vi "Untitled 7.vi"(0 "Tree":string(tree), 2 "Folder_Path":path=path "D:/Git/Assignments/Assignment-23", 11 "Error_In":errorcluster) -> (4 "Edit Tree Items:Add Item":string, 15 "Error_Out":errorcluster)   [LabVIEW 2023]
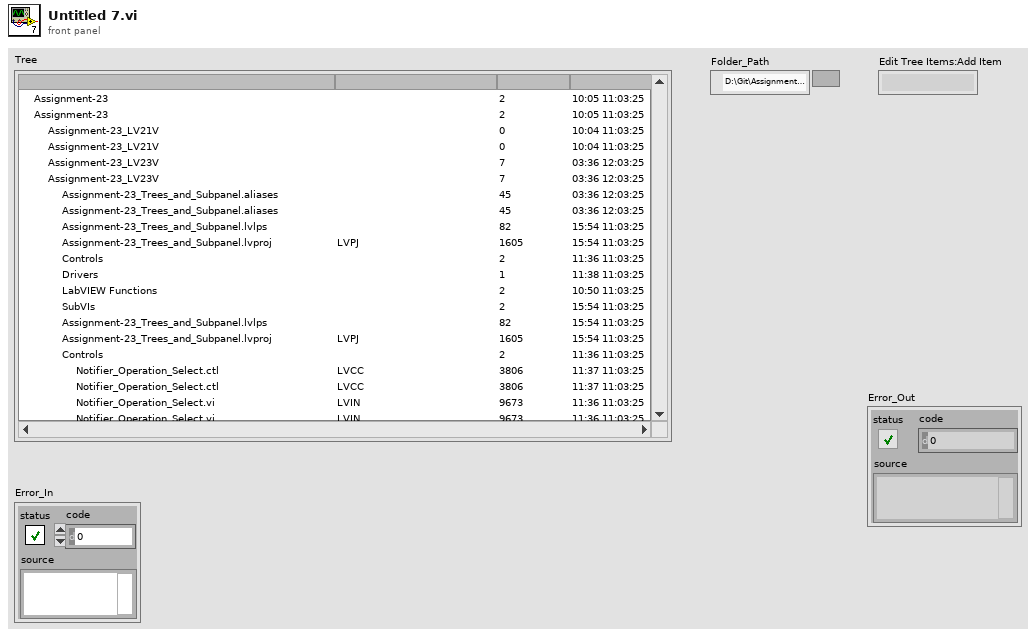
[diagram p1: front panel]
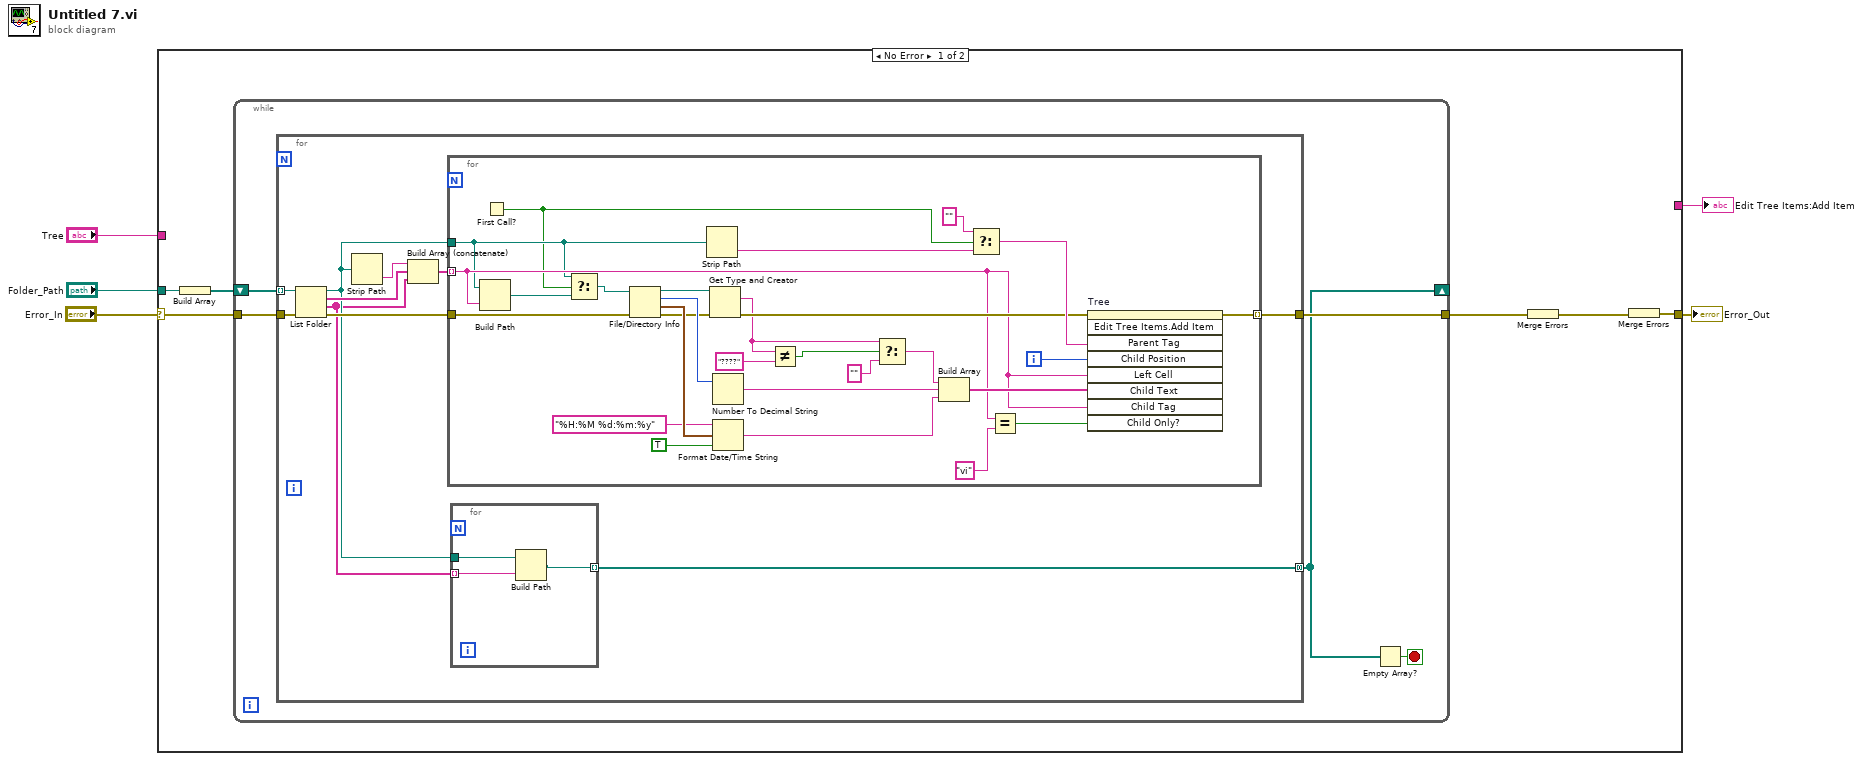
[diagram p0: block diagram]
diagram:
  n1 = case shown="No Error" "Error_In" {
    selector: "Error_In" -> [w11 w59]
    tunnel: "Folder_Path" -> [w10 _]
    tunnel: [w9 w59] -> w3
    tunnel: [_ w58] -> w2
    tunnel: "Tree" -> [_ w58]
    frame No Error {
      n2 = Build Array(w10) -> (w7:path[])
      n3 = while {
        tunnel: w11 -> [w16]
        tunnel: [w14] -> w6
        shift-right: [w13] -> _
        shift-left: w7 -> [w15]
        stop <- w12 stop-if-true
        n4 = for {
          tunnel: w16 -> [w26]
          tunnel: w15 -> [w25] mode=indexing
          tunnel: [w21] -> w14
          tunnel: [w17] -> w13 mode=concatenating
          n5 = List Folder(path=w25, error in=w26) -> (path out=w19:path, filenames=w23:string[], folder names=w18:string[], error out=w24:errorcluster)  [unwired: 2 in]
          n6 = Strip Path(path=w19) -> (name=w22:string)  [unwired: 1 out]
          n7 = Build Array (concatenate)(w22, w23, w18) -> (w20:string[])
          n8 = for {
            tunnel: w19 -> [w31]
            tunnel: w24 -> [w44]
            tunnel: [w43] -> w21 mode=indexing
            tunnel: w20 -> [w34] mode=indexing
            i -> [w47]
            n9 = Build Path(base path=w31, name or relative path=w34) -> (appended path=w33:path)
            n10 = First Call?() -> (First Call?: T/F=w30:bool)
            n11 = Select(t=w31, s=w30, f=w33) -> (s? t:f=w32:path)
            n12 = File/Directory Info(path=w32, error in=w44) -> (path out=w40:path, size=w56:i64, last mod=w57:timestamp, error out=w42:errorcluster)  [unwired: 3 out]
            n13 = Strip Path(path=w31) -> (name=w50:string)  [unwired: 1 out]
            n14 = Get Type and Creator(4:w42, 7:w40) -> (0:w41:errorcluster, 2:w37:string)  [unwired: 2 out]
            n15 = Number To Decimal String(number=w56) -> (decimal integer string=w55:string)  [unwired: 1 in]
            n16 = Format Date/Time String(time format string (%c)="%H:%M %d:%m:%y", seconds (now)=w57, UTC format=TRUE) -> (date/time string=w54:string)
            n17 = Not Equal?(x=w37, y="????") -> (x != y?=w35:bool)
            n18 = Select(t=w37, s=w35, f="") -> (s? t:f=w39:string)
            n19 = Build Array(w39, w55, w54) -> (w53:string[])
            n20 = Select(t="", s=w30, f=w50) -> (s? t:f=w46:string)
            n21 = Equal?(x=w34, y="vi") -> (x = y?=w48:bool)
            n22 = invoke on="Tree" class="Tree (strict)" method="Edit Tree Items.Add Item"(error in=w41, "Parent Tag"=w46, "Child Position"=w47, "Left Cell"=w34, "Child Text"=w53, "Child Tag"=w34, "Child Only?"=w48) -> (error out=w43:errorcluster)  [unwired: 2 in, 8 out]
          }
          n23 = for {
            tunnel: w19 -> [w29]
            tunnel: w18 -> [w28] mode=indexing
            tunnel: [w27] -> w17 mode=indexing
            n24 = Build Path(base path=w29, name or relative path=w28) -> (appended path=w27:path)
          }
        }
        n25 = Empty Array?(array=w13) -> (empty?=w12:bool)
      }
      n26 = Merge Errors(w6) -> (w8:errorcluster)
      n27 = Merge Errors(w8) -> (w9:errorcluster)
    }
    frame Error {
    }
  }
  "Error_Out" <- w3
  "Edit Tree Items:Add Item" <- w2
